vi "Get Tag Value from file.vi"(7 "Litt/BigEnd":bool, 8 "error in":errorcluster, 9 "Tag Code":u16, 10 "DirEntries":T1[](array[typedef]), 11 "File":refnum<file>) -> (0 "error out":errorcluster, 1 "Multiple Values":u64[](array[numeric]), 2 "Single Value":u32, 3 "File":refnum<file>, 4 "Array of Rationals":dbl[](array[numeric]), 5 "Tag exists?":bool)   [LabVIEW 2013, in "Tiff reader.lvlib"]
doc: "Reads a single specific tag in the array of tags returned by Read Image File Directory.vi and returns the associated data (either a single value or multiple values). The definition and meaning of the various tags is given in the tiff specifications."
uses:
  Tiff reader.lvlib
  IFD Entry.ctl
  FieldTypes.ctl
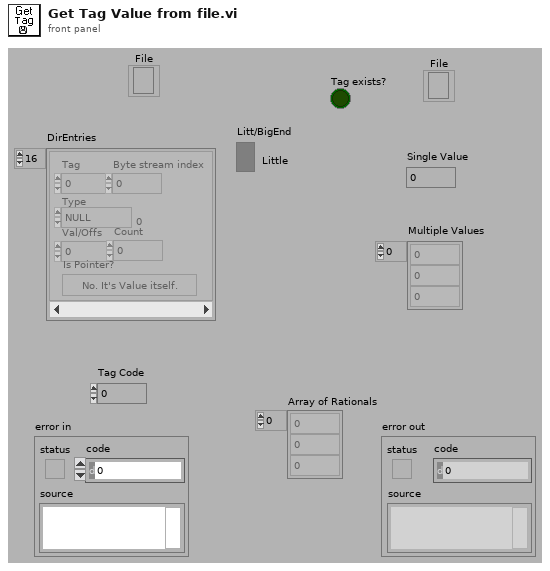
[diagram p1: front panel]
types:
  T1 = typedef "Tiff reader.lvlib/IFD Entry.ctl" = cluster{"Tag":u16, "Type":T2, "Count":u32, "Val/Offs":u32, "Is Pointer?":bool, "Byte stream index":i32}
  T2 = typedef "Tiff reader.lvlib/FieldTypes.ctl" = enum16{"NULL", "U8", "ASCII7", "U16", "U32", "RATIONAL", "SByte(I8)", "Undef(8Bit)", "I16", "I32", "SRat(4B:4B)", "SGL(4Byte)", "DBL(8Byte)"}
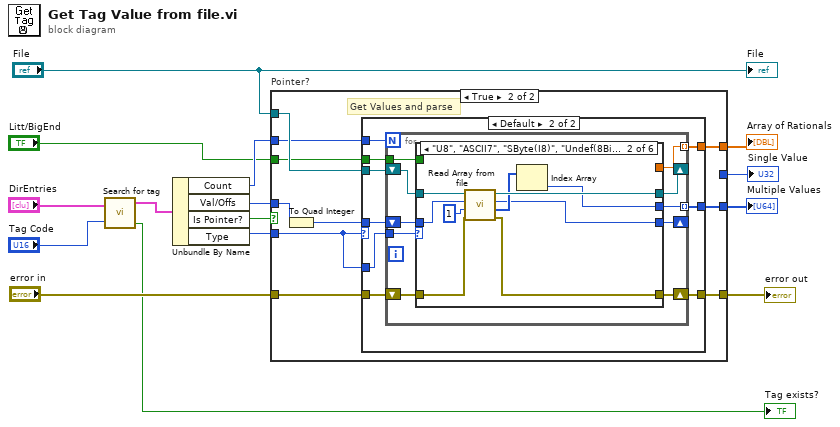
[diagram p0: block diagram]
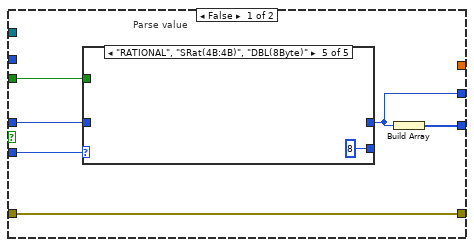
[diagram p2: hidden frame]
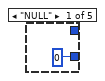
[diagram p3: hidden frame]
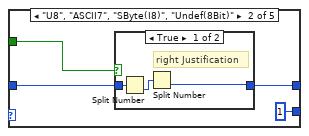
[diagram p4: hidden frame]
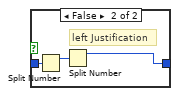
[diagram p5: hidden frame]
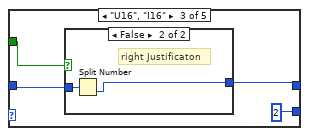
[diagram p6: hidden frame]
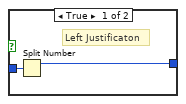
[diagram p7: hidden frame]
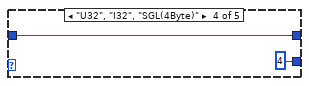
[diagram p8: hidden frame]
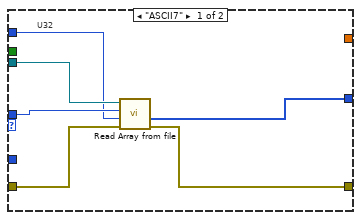
[diagram p9: hidden frame]
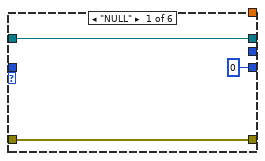
[diagram p10: hidden frame]
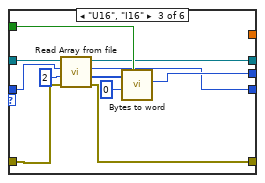
[diagram p11: hidden frame]
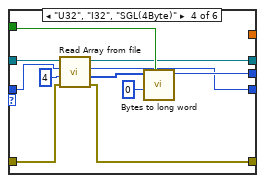
[diagram p12: hidden frame]
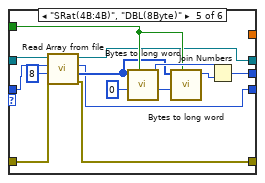
[diagram p13: hidden frame]
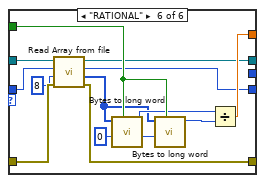
[diagram p14: hidden frame]
diagram:
  n1 = call "Search for tag.vi"("Directory"="DirEntries", "Tag"="Tag Code") -> ("Tag found"=w7:T1, "Tag exists?"=→"Tag exists?":bool)  [unwired: 1 out]
  n2 = Unbundle By Name(w7) -> ("Count"=w11:u32, "Val/Offs"=w14:u32, "Is Pointer?"=w15:bool, "Type"=w13:T2)
  n3 = case "Pointer?" shown="True" w15 {
    tunnel: w14 -> [w19 w52]
    tunnel: w13 -> [w20 w44]
    tunnel: "File" -> [_ w51]
    tunnel: [w21 w53] -> w12
    tunnel: w11 -> [_ w50]
    tunnel: [w18 _] -> w10
    tunnel: "Litt/BigEnd" -> [w17 w48]
    tunnel: [_ w47] -> w8
    tunnel: "error in" -> [w16 w46]
    tunnel: [w16 w45] -> w2
    frame False {
      # "Parse value"
      n4 = case shown="\"RATIONAL\", \"SRat(4B:4B)\", \"DBL(8Byte)\"" w20 {
        tunnel: [0 1 2 4 8] -> _
        tunnel: w19 -> [_ w25 w35 w41 _]
        tunnel: [_ w24 w34 w41 _] -> w18
        tunnel: w17 -> [_ w23 w33 _ _]
        frame "NULL" {
        }
        frame "U8", "ASCII7", "SByte(I8)", "Undef(8Bit)" {
          n5 = case shown="True" w23 {
            tunnel: w25 -> [w29 w32]
            tunnel: [w27 w30] -> w24
            frame True {
              # "right Justification"
              n6 = Split Number(x=w29) -> (lo(x)=w28:u16)  [unwired: 1 out]
              n7 = Split Number(x=w28) -> (lo(x)=w27:u8)  [unwired: 1 out]
            }
            frame False {
              # "left Justification"
              n8 = Split Number(x=w32) -> (hi(x)=w31:u16)  [unwired: 1 out]
              n9 = Split Number(x=w31) -> (hi(x)=w30:u8)  [unwired: 1 out]
            }
          }
        }
        frame "U16", "I16" {
          n10 = case shown="False" w33 {
            tunnel: w35 -> [w38 w40]
            tunnel: [w37 w39] -> w34
            frame True {
              # "Left Justificaton"
              n11 = Split Number(x=w38) -> (hi(x)=w37:u16)  [unwired: 1 out]
            }
            frame False {
              # "right Justificaton"
              n12 = Split Number(x=w40) -> (lo(x)=w39:u16)  [unwired: 1 out]
            }
          }
        }
        frame "U32", "I32", "SGL(4Byte)" {
        }
        frame "RATIONAL", "SRat(4B:4B)", "DBL(8Byte)" {
        }
      }
      n13 = Build Array(w18) -> (w21:u32[])
    }
    frame True {
      # "Get Values and parse"
      n14 = To Quad Integer(1:w52) -> (0:w49:i64)
      n15 = case shown="Default" w44 {
        tunnel: [w55 w68] -> w53
        tunnel: w51 -> [w59 w67]
        tunnel: w50 -> [w54 w66]
        tunnel: w49 -> [w57 w65]
        tunnel: w48 -> [_ w64]
        tunnel: [_ w63] -> w47
        tunnel: w46 -> [w58 w62]
        tunnel: [w56 w61] -> w45
        tunnel: w44 -> [_ w60]
        frame "ASCII7" {
          # "U32"
          n16 = call "Read Array from file.vi"("error in"=w58, "bytes to read"=w54, "File location in"=w57, "File"=w59) -> ("error out"=w56:errorcluster, "Array of U8s"=w55:u8[])  [unwired: 2 out]
        }
        frame Default {
          n17 = for {
            N: w66 -> [_]
            tunnel: w60 -> [w78]
            tunnel: [w76] -> w68 mode=indexing
            shift-right: [w74] -> _
            shift-left: w65 -> [w75]
            tunnel: w64 -> [w73]
            tunnel: [w72] -> w63 mode=indexing
            shift-right: [w71] -> _
            shift-left: w67 -> [w77]
            shift-right: [w70] -> w61
            shift-left: w62 -> [w69]
            n18 = case shown="\"U8\", \"ASCII7\", \"SByte(I8)\", \"Undef(8Bit)\"" w78 {
              tunnel: w77 -> [w80 w88 w99 w110 w121 w135]
              tunnel: w75 -> [_ w89 w93 w106 w118 w133]
              tunnel: [_ w85 w101 w112 w123 _] -> w76
              tunnel: [0 ("Index+2") w84 w95 w107 w119 w128] -> w74
              tunnel: w73 -> [_ _ w100 w111 w122 w139]
              tunnel: [_ _ _ _ _ w136] -> w72
              tunnel: [w80 w87 w98 w109 w114 w131] -> w71
              tunnel: [w79 w83 w91 w103 w116 w129] -> w70
              tunnel: w69 -> [w79 w82 w92 w104 w115 w132]
              frame "NULL" {
              }
              frame "U8", "ASCII7", "SByte(I8)", "Undef(8Bit)" {
                n19 = call "Read Array from file.vi"("error in"=w82, "bytes to read"=1, "File location in"=w89, "File"=w88) -> ("error out"=w83:errorcluster, "Array of U8s"=w86:u8[], "File location after array read"=w84:i64, "File out"=w87:refnum<file>)
                n20 = Index Array(array=w86) -> (element=w85:u8)  [unwired: 1 in]
              }
              frame "U16", "I16" {
                n21 = call "Read Array from file.vi"("error in"=w92, "bytes to read"=2, "File location in"=w93, "File"=w99) -> ("error out"=w91:errorcluster, "Array of U8s"=w97:u8[], "File location after array read"=w95:i64, "File out"=w98:refnum<file>)
                n22 = call "Bytes to word.vi"("Litt/BigEnd"=w100, "Index"=0, "Image Data in"=w97) -> ("Word"=w101:u16)  [unwired: 2 in, 4 out]
              }
              frame "U32", "I32", "SGL(4Byte)" {
                n23 = call "Read Array from file.vi"("error in"=w104, "bytes to read"=4, "File location in"=w106, "File"=w110) -> ("error out"=w103:errorcluster, "Array of U8s"=w108:u8[], "File location after array read"=w107:i64, "File out"=w109:refnum<file>)
                n24 = call "Bytes to long word.vi"("Litt/BigEnd"=w111, "Index"=0, "Image Data in"=w108) -> ("U32"=w112:u32)  [unwired: 6 out]
              }
              frame "SRat(4B:4B)", "DBL(8Byte)" {
                n25 = call "Read Array from file.vi"("error in"=w115, "bytes to read"=8, "File location in"=w118, "File"=w121) -> ("error out"=w116:errorcluster, "Array of U8s"=w120:u8[], "File location after array read"=w119:i64, "File out"=w114:refnum<file>)
                n26 = call "Bytes to long word.vi"("Litt/BigEnd"=w122, "Index"=0, "Image Data in"=w120) -> ("Index+4"=w126:i32, "U32"=w125:u32)  [unwired: 5 out]
                n27 = call "Bytes to long word.vi"("Litt/BigEnd"=w122, "Index"=w126, "Image Data in"=w120) -> ("U32"=w124:u32)  [unwired: 6 out]
                n28 = Join Numbers(hi=w125, lo=w124) -> ((hi.lo)=w123:u64)
              }
              frame "RATIONAL" {
                n29 = call "Read Array from file.vi"("error in"=w132, "bytes to read"=8, "File location in"=w133, "File"=w135) -> ("error out"=w129:errorcluster, "Array of U8s"=w127:u8[], "File location after array read"=w128:i64, "File out"=w131:refnum<file>)
                n30 = call "Bytes to long word.vi"("Litt/BigEnd"=w139, "Index"=0, "Image Data in"=w127) -> ("Index+4"=w140:i32, "U32"=w138:u32)  [unwired: 5 out]
                n31 = call "Bytes to long word.vi"("Litt/BigEnd"=w139, "Index"=w140, "Image Data in"=w127) -> ("U32"=w137:u32)  [unwired: 6 out]
                n32 = Divide(x=w138, y=w137) -> (x/y=w136:dbl)
              }
            }
          }
        }
      }
    }
  }
  "Multiple Values" <- w12
  "Single Value" <- w10
  "Array of Rationals" <- w8
  "error out" <- w2
  "File" <- "File"
